vi "Helper Loop.vi"(8 "error in (no error)":errorcluster, 11 "Signal Analysis in":refnum<class "Signal Analysis.lvclass">) -> ()   [LabVIEW 2020, in "Signal Analysis.lvlib" / "Signal Analysis.lvclass"]
uses:
  Signal Analysis.lvclass
  C:/Program Files/National Instruments/LabVIEW 2025/vi.lib/ActorFramework/Actor/Actor.lvclass
  UI/UI Root/UI Root/Frequency Metadata.ctl
  Helper Loop State.ctl
  <vilib>/Natan Biesmans/G2CPU GPU and CPU HPC Toolkit/G2CPU Libraries/Arrays/1DArray/u32/1D Array u32.lvclass
  C:/Program Files/National Instruments/LabVIEW 2025/vi.lib/Natan Biesmans/G2CPU GPU and CPU HPC Toolkit/G2CPU Libraries/Arrays/Array/Array Prototype.lvclass
  <vilib>/Natan Biesmans/G2CPU GPU and CPU HPC Toolkit/G2CPU Libraries/Arrays/2DArray/s16/2D Array s16.lvclass
  <vilib>/Utility/miscctls.llb/LVOffsetAndMultiplierTypeDef.ctl
  Program Files/National Instruments/LabVIEW 2025/examples/Natan Biesmans/G2CPU GPU and CPU HPC Toolkit/_Examples/UI Acceleration/Signal Density Plot Config.ctl
  Signal Analysis.lvclass/Signal Analysis.ctl
  Helper Loop Message.ctl
  Helper Loop Type.ctl
  Process Data.ctl
  <vilib>/Natan Biesmans/G2CPU GPU and CPU HPC Toolkit/G2CPU Libraries/Arrays/1DArray/s16/1D Array s16.lvclass
  UI/UI Root/UI Root/Signal Density Plot Data.ctl
  UI/UI Root/UI Root/FFT Plot Data.ctl
  <vilib>/ActorFramework/Actor/Actor.lvclass/Actor.ctl
  Application Manager/Application Manager Messages/Visualize FFT Msg/Visualize FFT Msg.lvclass/Visualize FFT Msg.ctl
  <vilib>/ActorFramework/Message Enqueuer/Message Enqueuer.lvclass/Message Enqueuer.ctl
  Application Manager/Application Manager Messages/Update Processing Metrics Msg/Update Processing Metrics Msg.lvclass/Update Processing Metrics Msg.ctl
  FFT Size.ctl
  Low Prio Rendering.ctl
  3b7c5731-3288-422e-9579-54a588a7c3cc.vi
  5c8155d3-63a1-46d8-b807-fae1af1e600c.vi
  05f40b7a-0676-44ad-acd9-391c165d43ca.vi
  60a2c10f-7ea4-4c19-9847-04cfdb7c7b1d.vi
  b3cef79f-9c71-4781-96f4-977c5153f233.vi
  4c400397-ccdf-494a-85b7-b802f87979ea.vi
  e15d3b19-6d2e-4512-b034-1ccceea2a302.vi
  0b159706-0337-4146-9fcf-a9429f3d28bc.vi
  d3b2aca6-c04a-43a5-ac15-5dcc80cfe7fb.vi
  3b7c5731-3288-422e-9579-54a588a7c3cc.vi/6197f869-f6d4-49b3-9b2c-cc979b422c2e.vi
  3b7c5731-3288-422e-9579-54a588a7c3cc.vi/a7e86dbb-b4c0-485c-89c5-522e60ee265c.vi
  5c8155d3-63a1-46d8-b807-fae1af1e600c.vi/ff52a514-0e94-4685-9782-cee11f20a7e4.vi
  5c8155d3-63a1-46d8-b807-fae1af1e600c.vi/09f95493-deb6-40ba-ba08-e63bad1f3c71.vi
  05f40b7a-0676-44ad-acd9-391c165d43ca.vi/b1821858-f795-4172-8d77-0d2b0bdabb59.vi
  05f40b7a-0676-44ad-acd9-391c165d43ca.vi/d461e1dd-3ff8-4523-95b7-3ce56130f115.vi
  60a2c10f-7ea4-4c19-9847-04cfdb7c7b1d.vi/ef94ed2d-c4e6-48dc-8bdb-249d71a97973.vi
  b3cef79f-9c71-4781-96f4-977c5153f233.vi/ef94ed2d-c4e6-48dc-8bdb-249d71a97973.vi
  <vilib>/ActorFramework/Message Enqueuer/Enqueue.vi
  e15d3b19-6d2e-4512-b034-1ccceea2a302.vi/ab6cfe59-c8ad-4da3-839b-8d02ec9e015f.vi
  0b159706-0337-4146-9fcf-a9429f3d28bc.vi/46771f49-eb1d-473b-8e81-f516cef50a4e.vi
  0b159706-0337-4146-9fcf-a9429f3d28bc.vi/dc76f8e4-64fa-456a-8549-7a4b6936c4c9.vi
  0b159706-0337-4146-9fcf-a9429f3d28bc.vi/7e60ddfb-e748-4c0c-85da-e395a1b7978d.vi
  0b159706-0337-4146-9fcf-a9429f3d28bc.vi/d2eceff7-f641-4ce4-acfa-e9e293a3c877.vi
  0b159706-0337-4146-9fcf-a9429f3d28bc.vi/b737122b-4036-448b-abd3-e2701355e828.vi
  d3b2aca6-c04a-43a5-ac15-5dcc80cfe7fb.vi/e7247370-a01f-465a-ac0e-4dfefcb1bb87.vi
  d3b2aca6-c04a-43a5-ac15-5dcc80cfe7fb.vi/345e91f0-9a5e-4de4-af9c-133346717e4a.vi
  3b7c5731-3288-422e-9579-54a588a7c3cc.vi/6197f869-f6d4-49b3-9b2c-cc979b422c2e.vi/87b81512-7a6a-4bb0-93b2-4564eba18751.vi
  3b7c5731-3288-422e-9579-54a588a7c3cc.vi/6197f869-f6d4-49b3-9b2c-cc979b422c2e.vi/3b85cfcd-f2e7-425d-bf63-d84251333cff.vi
  3b7c5731-3288-422e-9579-54a588a7c3cc.vi/6197f869-f6d4-49b3-9b2c-cc979b422c2e.vi/bdde7ba0-fc5a-4512-a8ec-1695e5fcee25.vi
  3b7c5731-3288-422e-9579-54a588a7c3cc.vi/6197f869-f6d4-49b3-9b2c-cc979b422c2e.vi/3e802c67-fb96-46a3-ae13-4994a8508b4f.vi
  3b7c5731-3288-422e-9579-54a588a7c3cc.vi/6197f869-f6d4-49b3-9b2c-cc979b422c2e.vi/5a50fc67-79e7-4972-80c2-92243cd53dd4.vi
  3b7c5731-3288-422e-9579-54a588a7c3cc.vi/a7e86dbb-b4c0-485c-89c5-522e60ee265c.vi/730f6c57-5c0b-4ee9-b61e-75067b25222b.vi
  3b7c5731-3288-422e-9579-54a588a7c3cc.vi/a7e86dbb-b4c0-485c-89c5-522e60ee265c.vi/096b8799-7810-404e-baca-ba9279cec4bd.vi
  3b7c5731-3288-422e-9579-54a588a7c3cc.vi/a7e86dbb-b4c0-485c-89c5-522e60ee265c.vi/0f1a5a47-bcc5-4796-ac31-8dfcfbc0d7d1.vi
  3b7c5731-3288-422e-9579-54a588a7c3cc.vi/a7e86dbb-b4c0-485c-89c5-522e60ee265c.vi/89f12e17-3330-4b72-ad8f-8dd636660732.vi
  e15d3b19-6d2e-4512-b034-1ccceea2a302.vi/ab6cfe59-c8ad-4da3-839b-8d02ec9e015f.vi/313ec8c5-c203-475c-9de0-0583f6fb8b4d.vi
  0b159706-0337-4146-9fcf-a9429f3d28bc.vi/dc76f8e4-64fa-456a-8549-7a4b6936c4c9.vi/2c12aba4-aacf-4d7a-adbe-039f6155a93e.vi
  0b159706-0337-4146-9fcf-a9429f3d28bc.vi/dc76f8e4-64fa-456a-8549-7a4b6936c4c9.vi/f38cccb2-46f6-49f0-a8d6-9da0c88ff6f3.vi
  0b159706-0337-4146-9fcf-a9429f3d28bc.vi/dc76f8e4-64fa-456a-8549-7a4b6936c4c9.vi/bdde7ba0-fc5a-4512-a8ec-1695e5fcee25.vi
  0b159706-0337-4146-9fcf-a9429f3d28bc.vi/dc76f8e4-64fa-456a-8549-7a4b6936c4c9.vi/3e802c67-fb96-46a3-ae13-4994a8508b4f.vi
  0b159706-0337-4146-9fcf-a9429f3d28bc.vi/dc76f8e4-64fa-456a-8549-7a4b6936c4c9.vi/5a50fc67-79e7-4972-80c2-92243cd53dd4.vi
  3b7c5731-3288-422e-9579-54a588a7c3cc.vi/6197f869-f6d4-49b3-9b2c-cc979b422c2e.vi/3e802c67-fb96-46a3-ae13-4994a8508b4f.vi/1b7cf390-2ae0-48f3-9bce-03c57eed6ee8.vi
  0b159706-0337-4146-9fcf-a9429f3d28bc.vi/dc76f8e4-64fa-456a-8549-7a4b6936c4c9.vi/5a50fc67-79e7-4972-80c2-92243cd53dd4.vi/1b7cf390-2ae0-48f3-9bce-03c57eed6ee8.vi
  <vilib>/Natan Biesmans/G2CPU GPU and CPU HPC Toolkit/G2CPU Libraries/Arrays/1DArray/f32/1D Array f32.lvclass
  <vilib>/Natan Biesmans/G2CPU GPU and CPU HPC Toolkit/G2CPU Libraries/Arrays/2DArray/c32/2D Array c32.lvclass
  <vilib>/Natan Biesmans/G2CPU GPU and CPU HPC Toolkit/G2CPU Libraries/Arrays/2DArray/f32/2D Array f32.lvclass
  Application Manager/Application Manager Messages/Visualize FFT Msg/Visualize FFT Msg.lvclass
  C:/Program Files/National Instruments/LabVIEW 2025/vi.lib/ActorFramework/Message/Message.lvclass
  Application Manager/Application Manager Messages/Update Processing Metrics Msg/Update Processing Metrics Msg.lvclass
  <vilib>/Natan Biesmans/G2CPU GPU and CPU HPC Toolkit/G2CPU Libraries/Arrays/1DArray/u64/1D Array u64.lvclass
  <vilib>/Natan Biesmans/G2CPU GPU and CPU HPC Toolkit/ArrayFire Driver/VIs/Run as Multi Device.vi
  <vilib>/Natan Biesmans/G2CPU GPU and CPU HPC Toolkit/G2CPU Libraries/Manage Environment/Find AF DLL.vi
  <vilib>/Natan Biesmans/G2CPU GPU and CPU HPC Toolkit/ArrayFire Driver/subvi/Error Converter (ErrCode or Status).vi
  <vilib>/Natan Biesmans/G2CPU GPU and CPU HPC Toolkit/G2CPU Libraries/Arrays/Array/G2CPU Set Array Pointer.vi
  <vilib>/Natan Biesmans/G2CPU GPU and CPU HPC Toolkit/G2CPU Libraries/Arrays/Array/G2CPU Get Array Pointer.vi
  <vilib>/Natan Biesmans/G2CPU GPU and CPU HPC Toolkit/ArrayFire Driver/VIs/cast.vi
  <vilib>/Natan Biesmans/G2CPU GPU and CPU HPC Toolkit/G2CPU Libraries/Arrays/SubVI/Lock Arrays.vi
  <vilib>/Natan Biesmans/G2CPU GPU and CPU HPC Toolkit/G2CPU Libraries/Arrays/SubVI/is 2D.vi
  <vilib>/Natan Biesmans/G2CPU GPU and CPU HPC Toolkit/ArrayFire Driver/VIs/mul.vi
  <vilib>/Natan Biesmans/G2CPU GPU and CPU HPC Toolkit/G2CPU Libraries/Arrays/Array/G2CPU Unlock Array.vi
  <vilib>/Natan Biesmans/G2CPU GPU and CPU HPC Toolkit/ArrayFire Driver/VIs/fft inplace.vi
  <vilib>/Natan Biesmans/G2CPU GPU and CPU HPC Toolkit/ArrayFire Driver/VIs/max by key.vi
  <vilib>/Natan Biesmans/G2CPU GPU and CPU HPC Toolkit/G2CPU Libraries/Arrays/Array/G2CPU Get Array Size.vi
  <vilib>/Natan Biesmans/G2CPU GPU and CPU HPC Toolkit/G2CPU Libraries/Arrays/Array/G2CPU Get Data Type.vi
  <vilib>/Natan Biesmans/G2CPU GPU and CPU HPC Toolkit/ArrayFire Driver/VIs/is scalar.vi
  <vilib>/Natan Biesmans/G2CPU GPU and CPU HPC Toolkit/ArrayFire Driver/VIs/is empty.vi
  <vilib>/ActorFramework/Message Priority Queue/Priority Enqueue.vi
  <vilib>/Natan Biesmans/G2CPU GPU and CPU HPC Toolkit/ArrayFire Driver/VIs/range.vi
  <vilib>/Natan Biesmans/G2CPU GPU and CPU HPC Toolkit/G2CPU Libraries/Arrays/SubVI/is 1D.vi
  <vilib>/Natan Biesmans/G2CPU GPU and CPU HPC Toolkit/ArrayFire Driver/VIs/div.vi
  <vilib>/Natan Biesmans/G2CPU GPU and CPU HPC Toolkit/G2CPU Libraries/Arrays/Array/Array Prototype.lvclass
  <vilib>/Natan Biesmans/G2CPU GPU and CPU HPC Toolkit/G2CPU Libraries/Arrays/DataTypes/c32/c32.lvclass
  <vilib>/Natan Biesmans/G2CPU GPU and CPU HPC Toolkit/G2CPU Libraries/Arrays/2DArray/2D Array Prototype.lvclass
  <vilib>/Natan Biesmans/G2CPU GPU and CPU HPC Toolkit/G2CPU Libraries/Arrays/DataTypes/f32/f32.lvclass
  <vilib>/Natan Biesmans/G2CPU GPU and CPU HPC Toolkit/G2CPU Libraries/Arrays/1DArray/1D Array Prototype.lvclass
  <vilib>/ptbypt/NI_PtbyPt.lvlib
  <vilib>/Natan Biesmans/G2CPU GPU and CPU HPC Toolkit/G2CPU Libraries/UI Acceleration/G2CPU Signal Density Plots.lvlib
  UI/UI Root/UI Root/UI Root.lvclass
  <vilib>/ActorFramework/Actor/Actor.lvclass
panel:
  in  "Frequency Metedata":T1
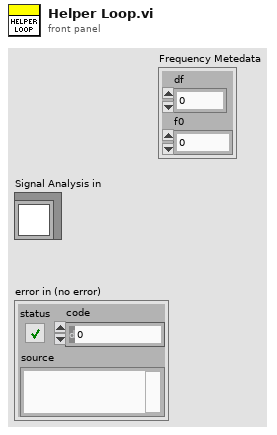
[diagram p1: front panel]
types:
  T1 = typedef "UI Root.lvlib/UI Root.lvclass/Frequency Metadata.ctl" = cluster{"df":dbl, "f0":dbl}
  T2 = typedef "Signal Analysis.lvlib/Signal Analysis.lvclass/Helper Loop State.ctl" = cluster{"First Run":bool, "Plot Scale":cluster{"X Scale":T3, "Y Scale":T3}, "Predefined Configuration Parameters":cluster{"Column Counter":refnum<class "1D Array u32.lvclass">, "Full Bin Range":refnum<class "2D Array s16.lvclass">}, "FFT Size":i32, "Low Prio Rendering":bool, "FFT Scaling Map":refnum<class "1D Array u32.lvclass">, "FFT Scaling":dbl, "Graph Config":T4}
  T3 = typedef "LVOffsetAndMultiplierTypeDef.ctl" = cluster{"Offset":dbl, "Multiplier":dbl}
  T4 = typedef "G2CPU Signal Density Plots.lvlib/Signal Density Plot Config.ctl" = cluster{"X resolution":u64, "Y resolution":u64, "Min":sgl, "Max":sgl}
  T5 = typedef "UI Root.lvlib/UI Root.lvclass/FFT Plot Data.ctl" = cluster{"FFT":refnum<data-value>, "Scaling":dbl, "Raw FFT Size":i32}
  T6 = typedef "UI Root.lvlib/UI Root.lvclass/Signal Density Plot Data.ctl" = cluster{"Plot":refnum<data-value>, "Plot Scale":cluster{"X Scale":T3, "Y Scale":T3}}
  T7 = typedef "Signal Analysis.lvlib/Signal Analysis.lvclass/Process Data.ctl" = cluster{"Gain":dbl, "dt":dbl, "Serial IQ Data":refnum<class "1D Array s16.lvclass">, "f0":dbl}
  T8 = typedef "Signal Analysis.lvlib/Signal Analysis.lvclass/FFT Size.ctl" = cluster{"FFT Size":i32}
  T9 = typedef "Signal Analysis.lvlib/Signal Analysis.lvclass/Low Prio Rendering.ctl" = cluster{"Low Prio Rendering":bool}
  T10 = typedef "Signal Analysis.lvlib/Signal Analysis.lvclass/Helper Loop Message.ctl" = cluster{"Type":T11, "Payload":variant}
  T11 = typedef "Signal Analysis.lvlib/Signal Analysis.lvclass/Helper Loop Type.ctl" = enum16{"Process Data", "Set Batch Size", "Set Render Prio", "Close", "Set FFT Size"}
  T12 = cluster{"Column Counter":refnum<class "1D Array u32.lvclass">, "Full Bin Range":refnum<class "2D Array s16.lvclass">}
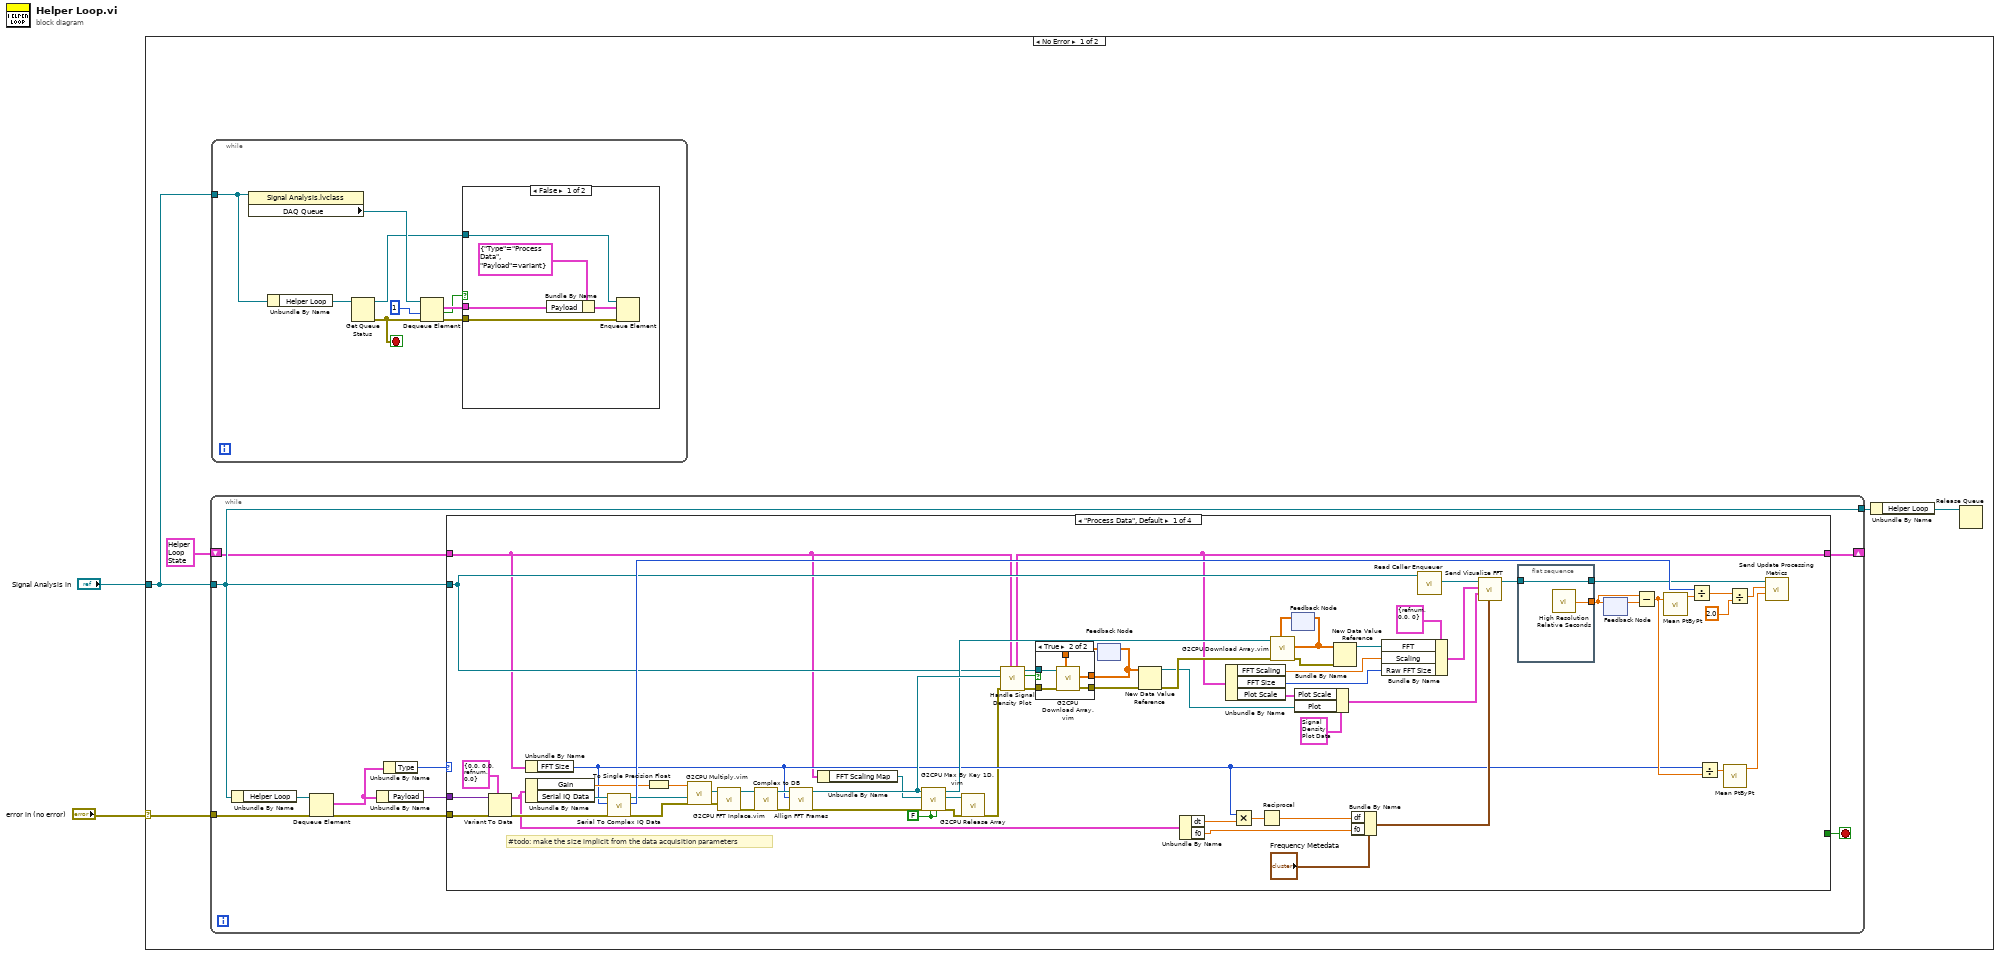
[diagram p0: block diagram]
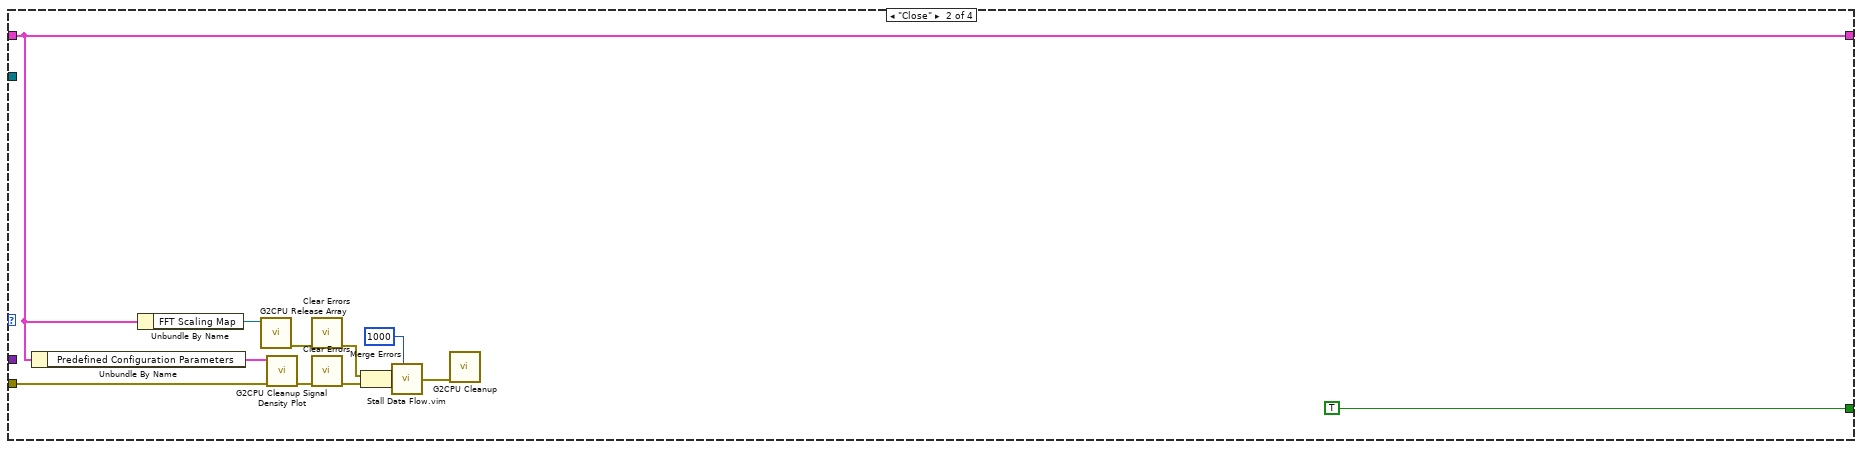
[diagram p3: hidden frame]
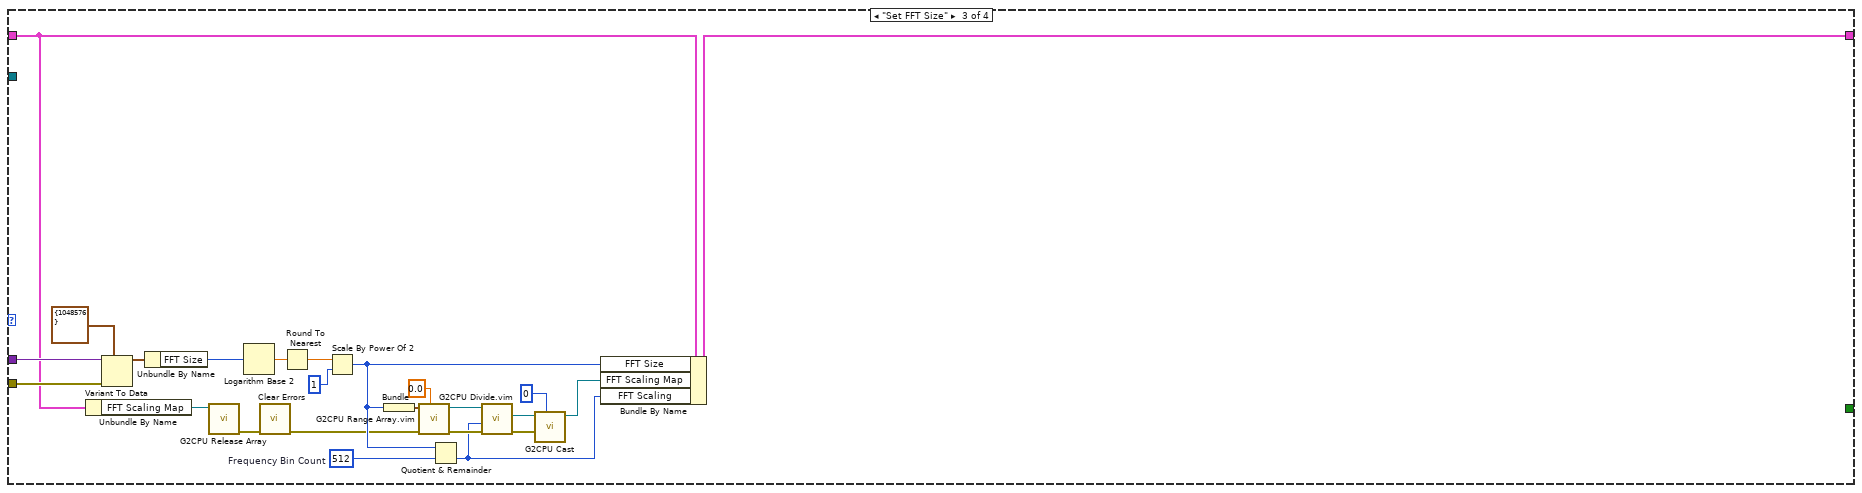
[diagram p4: hidden frame]
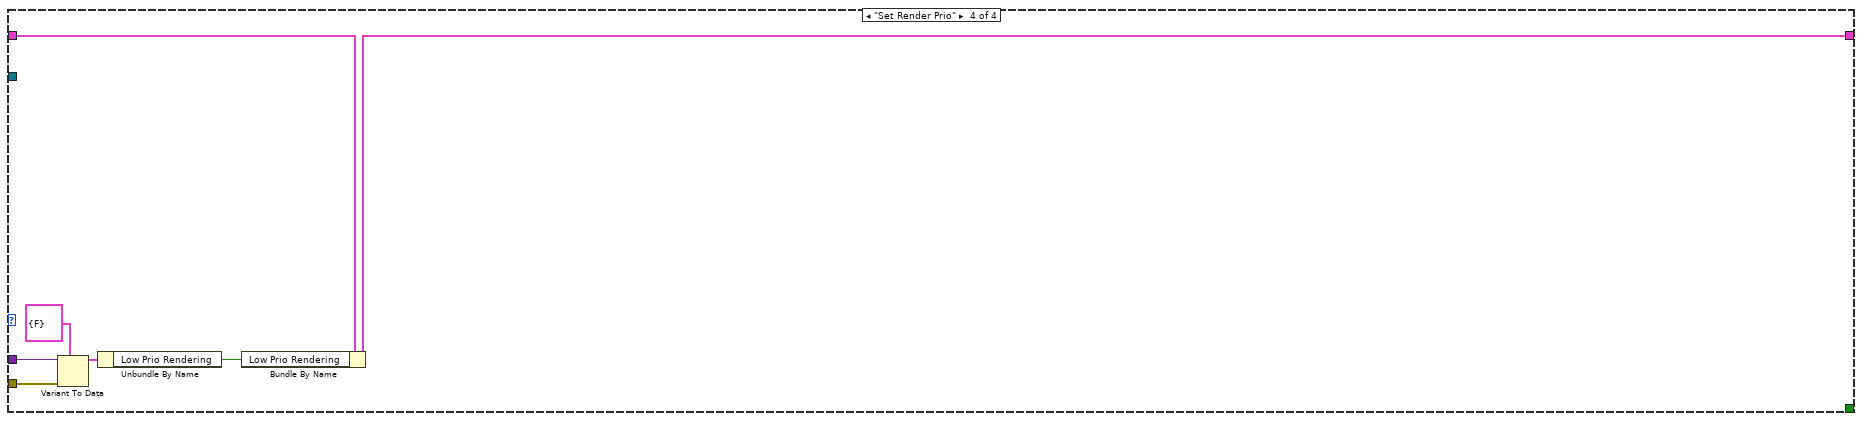
[diagram p5: hidden frame]
diagram:
  n1 = case shown="No Error" "error in (no error)" {
    selector: "error in (no error)" -> [w7 _]
    tunnel: "Signal Analysis in" -> [w6 _]
    frame No Error {
      n2 = while {
        tunnel: w6 -> [w12]
        tunnel: w7 -> [w17]
        tunnel: [w12] -> w5
        shift-right: [w9] -> _
        shift-left: T2 {"First Run"=TRUE, "Plot Scale"={"X Scale"={"Offset"=0.0, "Multiplier"=0.0}, "Y Scale"={"Offset"=0.0, "Multiplier"=0.0}}, "Predefined Configuration Parameters"={"Column Counter"=refnum, "Full Bin Range"=refnum}, "FFT Size"=1048576, "Low Prio Rendering"=FALSE, "FFT Scaling Map"=refnum, "FFT Scaling"=0.0, "Graph Config"={"X resolution"=0, "Y resolution"=0, "Min"=0.0, "Max"=0.0}} ("State") -> [w8]
        stop <- w14 stop-if-true
        n3 = Unbundle By Name(w12) -> ("Helper Loop"=w16:refnum<queue>)
        n4 = Dequeue Element(queue=w16, error in (no error)=w17) -> (element=w13:T10, error out=w15:errorcluster)  [unwired: 1 in, 2 out]
        n5 = Unbundle By Name(w13) -> ("Payload"=w10:variant)
        n6 = Unbundle By Name(w13) -> ("Type"=w11:T11)
        n7 = case shown="\"Process Data\", Default" w11 {
          tunnel: w12 -> [w40 _ _ _]
          tunnel: w15 -> [w83 w103 w126 w134]
          tunnel: [_ TRUE _ _] -> w14
          tunnel: w10 -> [w82 _ w127 w133]
          tunnel: [w30 w95 w128 w131] -> w9
          tunnel: w8 -> [w31 w95 w110 w135]
          frame "Process Data", Default {
            w36 = FALSE ("Auto Release Keys (Enabled)")
            # "#todo: make the size implicit from the data acquisition parameters"
            n8 = Variant To Data(error in=w83, type=T7 {"Gain"=0.0, "dt"=0.0, "Serial IQ Data"=refnum, "f0"=0.0} ("Filled Buffers"), Variant=w82) -> (data=w50:T7, error out=w81:errorcluster)
            n9 = Unbundle By Name(w50) -> ("Gain"=w56:dbl, "Serial IQ Data"=w61:refnum<class "1D Array s16.lvclass">)
            n10 = Unbundle By Name(w31) -> ("FFT Size"=w39:i32)
            n11 = call "Serial To Complex IQ Data.vi"("error in (no error)"=w81, "FFT Size"=w39, "Serial Data In"=w61) -> ("error out"=w53:errorcluster, "Amount Of Samples"=w74:u64, "Batched Complex Data Out"=w55:refnum<class "2D Array c32.lvclass">)  [unwired: 5 in, 1 out]
            n12 = To Single Precision Float(number=w56) -> (single precision float=w54:sgl)
            n13 = call "G2CPU Multiply.vim"("error in (no error)"=w53, "Array rhs"=w55, "Array lhs"=w54) -> ("error out"=w52:errorcluster, "Array Result"=w51:refnum<class "2D Array c32.lvclass">)  [unwired: 7 in]
            n14 = call "G2CPU FFT Inplace.vim"("error in (no error)"=w52, "Array Signal"=w51) -> ("error out"=w57:errorcluster, "Array out"=w58:refnum<class "2D Array c32.lvclass">)  [unwired: 8 in]
            n15 = call "Complex to DB.vi"("error in (no error)"=w57, "Complix FFT In"=w58) -> ("error out"=w59:errorcluster, "Db Amplitude Out"=w60:refnum<class "2D Array f32.lvclass">)  [unwired: 8 in]
            n16 = call "Allign FFT Frames.vi"("error in (no error)"=w59, "FFT Size"=w39, "FFT Frame in"=w60) -> ("error out"=w38:errorcluster, "Alligned FFT Frame Out"=w65:refnum<class "2D Array f32.lvclass">)  [unwired: 6 in, 1 out]
            n17 = Unbundle By Name(w31) -> ("FFT Scaling Map"=w37:refnum<class "1D Array u32.lvclass">)
            n18 = call "G2CPU Max By Key 1D.vim"("Auto Release Keys (Enabled)"=w36, "Auto Release Array In (Enabled)"=w36, "error in (no error)"=w38, "Array Keys 1D U32"=w37, "Array"=w65) -> ("error out"=w79:errorcluster, "Array Keys"=w80:refnum<class "1D Array u32.lvclass">, "Array out"=w41:refnum<class "2D Array f32.lvclass">)  [unwired: 4 in]
            n19 = call <vilib>:"G2CPU Release Array.vi"("error in (no error)"=w79, "Array in"=w80) -> ("error out"=w32:errorcluster)  [unwired: 9 in]
            n20 = call "Handle Signal Density Plot.vi"("State in"=w31, "error in (no error)"=w32, "Alligned FFT Frame Out"=w65, "Signal Analysis in"=w40) -> ("error out"=w70:errorcluster, "Signal Density Plot Available"=w29:bool, "Signal Density Plot"=w69:refnum<class "2D Array f32.lvclass">, "State out"=w30:T2)  [unwired: 4 in]
            n21 = feedback #1() -> (w68:sgl[][])  [unwired: 1 in]
            n22 = case shown="True" w29 {
              tunnel: w70 -> [w86 w92]
              tunnel: w69 -> [_ w91]
              tunnel: w68 -> [w87 w90]
              tunnel: [w86 w89] -> w67
              tunnel: [w87 w88] -> w66
              frame False {
              }
              frame True {
                n23 = call "G2CPU Download Array.vim"("Pre Allocated Buffer"=w90, "error in (no error)"=w92, "Array in"=w91) -> ("error out"=w89:errorcluster, "Array Data"=w88:sgl[][])  [unwired: 6 in, 1 out]
              }
            }
            n24 = feedback-in #1(w66) -> ()
            n25 = New Data Value Reference(data value=w66, error in=w67) -> (data value reference=w28:refnum<data-value>, error out=w42:errorcluster)
            n26 = Unbundle By Name(w50) -> ("dt"=w49:dbl, "f0"=w33:dbl)
            n27 = Unbundle By Name(w30) -> ("FFT Scaling"=w35:dbl, "FFT Size"=w34:i32, "Plot Scale"=w27:cluster{"X Scale":T3, "Y Scale":T3})
            n28 = Multiply(x=w39, y=w49) -> (x*y=w44:dbl)
            n29 = Reciprocal(x=w44) -> (1/x=w43:dbl)
            n30 = feedback #2() -> (w26:sgl[][])  [unwired: 1 in]
            n31 = call "G2CPU Download Array.vim"("Pre Allocated Buffer"=w26, "error in (no error)"=w42, "Array in"=w41) -> ("error out"=w21:errorcluster, "Array Data"=w25:sgl[][])  [unwired: 6 in, 1 out]
            n32 = feedback-in #2(w25) -> ()
            n33 = Bundle By Name(cluster=T6 {"Plot"=refnum, "Plot Scale"={"X Scale"={"Offset"=0.0, "Multiplier"=0.0}, "Y Scale"={"Offset"=0.0, "Multiplier"=0.0}}} ("output cluster 2"), "Plot Scale"=w27, "Plot"=w28) -> (w47:T6)
            n34 = New Data Value Reference(data value=w25, error in=w21) -> (data value reference=w22:refnum<data-value>)  [unwired: 1 out]
            n35 = Bundle By Name(cluster="Frequency Metedata", "df"=w43, "f0"=w33) -> (w45:T1)
            n36 = Bundle By Name(cluster=T5 {"FFT"=refnum, "Scaling"=0.0, "Raw FFT Size"=0} ("FFT Data"), "FFT"=w22, "Scaling"=w35, "Raw FFT Size"=w34) -> (w23:T5)
            n37 = call <vilib>:"Read Caller Enqueuer.vi"("Actor"=w40) -> ("Caller Enqueuer"=w20:refnum<class "Message Enqueuer.lvclass">)  [unwired: 10 in]
            n38 = call "Send Visualize FFT.vi"("Frequency Metedata"=w45, "Signal Density Plot"=w47, "FFT Data"=w23, "Message Enqueuer"=w20) -> ("Message Enqueuer out"=w19:refnum<class "Message Enqueuer.lvclass">)  [unwired: 6 in, 1 out]
            n39 = flat-sequence {
              tunnel: [w85] -> w77
              tunnel: [w84] -> w18
              tunnel: w19 -> [w84]
              frame #0 {
                n40 = call <vilib>:"High Resolution Relative Seconds.vi"() -> ("relative seconds"=w85:dbl)
              }
            }
            n41 = feedback #3() -> (w78:dbl)  [unwired: 1 in]
            n42 = feedback-in #3(w77) -> ()
            n43 = Subtract(x=w77, y=w78) -> (x-y=w72:dbl)
            n44 = call <vilib>:"Mean PtByPt.vi"("x"=w72) -> ("mean"=w76:dbl)  [unwired: 3 in, 1 out]
            n45 = Divide(x=w74, y=w76) -> (x/y=w75:dbl)
            n46 = Divide(x=w39, y=w72) -> (x/y=w71:dbl)
            n47 = call <vilib>:"Mean PtByPt.vi"("x"=w71) -> ("mean"=w64:dbl)  [unwired: 3 in, 1 out]
            n48 = Divide(x=w75, y=2.0) -> (x/y=w63:dbl)
            n49 = call "Send Update Processing Metrics.vi"("Peak Output"=w64, "System Throughput"=w63, "Message Enqueuer"=w18) -> ()  [unwired: 7 in, 2 out]
          }
          frame "Close" {
            n50 = Unbundle By Name(w95) -> ("Predefined Configuration Parameters"=w98:T12)
            n51 = Unbundle By Name(w95) -> ("FFT Scaling Map"=w97:refnum<class "1D Array u32.lvclass">)
            n52 = call <vilib>:"G2CPU Release Array.vi"("Array in"=w97) -> ("error out"=w96:errorcluster)  [unwired: 10 in]
            n53 = call <vilib>:"G2CPU Cleanup Signal Density Plot.vi"("error in (no error)"=w103, "Predefined Configuration Parameters"=w98) -> ("error out"=w100:errorcluster)  [unwired: 9 in]
            n54 = call <vilib>:"Clear Errors.vi"("error in (no error)"=w96) -> ("error out"=w93:errorcluster)  [unwired: 5 in, 1 out]
            n55 = call <vilib>:"Clear Errors.vi"("error in (no error)"=w100) -> ("error out"=w99:errorcluster)  [unwired: 5 in, 1 out]
            n56 = Merge Errors(w93, w99) -> (w94:errorcluster)
            n57 = call "Stall Data Flow.vim"("value in"=w94, "milliseconds to wait"=u32 1000) -> ("value out"=w102:errorcluster)  [unwired: 1 out]
            n58 = call <vilib>:"G2CPU Cleanup.vi"("error in (no error)"=w102) -> ()  [unwired: 10 in, 1 out]
          }
          frame "Set FFT Size" {
            w106 = u64 512  # Frequency Bin Count
            n59 = Unbundle By Name(w110) -> ("FFT Scaling Map"=w109:refnum<class "1D Array u32.lvclass">)
            n60 = Variant To Data(error in=w126, type=T8 {"FFT Size"=1048576} ("FFT Size"), Variant=w127) -> (data=w124:T8)  [unwired: 1 out]
            n61 = Unbundle By Name(w124) -> ("FFT Size"=w120:i32)
            n62 = call <vilib>:"G2CPU Release Array.vi"("Array in"=w109) -> ("error out"=w108:errorcluster)  [unwired: 10 in]
            n63 = Logarithm Base 2(1:w120) -> (0:w123:dbl)
            n64 = call <vilib>:"Clear Errors.vi"("error in (no error)"=w108) -> ("error out"=w107:errorcluster)  [unwired: 5 in, 1 out]
            n65 = Round To Nearest(number=w123) -> (nearest integer value=w122:dbl)
            n66 = Scale By Power Of 2(n=w122, x=u64 1) -> (x*2^n=w112:u64)
            n67 = Bundle(w112) -> (w119:cluster{u64})  [unwired: 1 in]
            n68 = call "G2CPU Range Array.vim"("Datatype"=sgl 0.0, "Error in"=w107, "Size"=w119) -> ("error out"=w116:errorcluster, "Array out"=w115:refnum<class "1D Array f32.lvclass">)  [unwired: 7 in]
            n69 = Quotient & Remainder(x=w112, y=w106) -> (floor(x/y)=w105:u64)  [unwired: 1 out]
            n70 = call "G2CPU Divide.vim"("error in (no error)"=w116, "Array rhs"=w105, "Array lhs"=w115) -> ("error out"=w118:errorcluster, "Array Result"=w117:refnum<class "1D Array f32.lvclass">)  [unwired: 7 in]
            n71 = call "G2CPU Cast"("Datatype Prototype"=u32 0, "error in (no error)"=w118, "Array In"=w117) -> ("Array Out"=w111:refnum<class "1D Array u32.lvclass">)  [unwired: 7 in, 1 out]
            n72 = Bundle By Name(cluster=w110, "FFT Size"=w112, "FFT Scaling Map"=w111, "FFT Scaling"=w105) -> (w128:T2)
          }
          frame "Set Render Prio" {
            n73 = Variant To Data(error in=w134, type=T9 {"Low Prio Rendering"=FALSE} ("Low Prio Rendering"), Variant=w133) -> (data=w130:T9)  [unwired: 1 out]
            n74 = Unbundle By Name(w130) -> ("Low Prio Rendering"=w129:bool)
            n75 = Bundle By Name(cluster=w135, "Low Prio Rendering"=w129) -> (w131:T2)
          }
        }
      }
      n76 = while {
        tunnel: w6 -> [w139]
        stop <- w138 stop-if-true
        n77 = property class="Signal Analysis.lvclass"(reference=w139) -> ("DAQ Queue"=w140:refnum<queue>)  [unwired: 1 in, 2 out]
        n78 = Unbundle By Name(w139) -> ("Helper Loop"=w137:refnum<queue>)
        n79 = Get Queue Status(queue=w137) -> (queue out=w136:refnum<queue>, error out=w138:errorcluster)  [unwired: 2 in, 6 out]
        n80 = Dequeue Element(queue=w140, timeout in ms (-1)=1, error in (no error)=w138) -> (element=w144:T7, timed out?=w143:bool, error out=w142:errorcluster)  [unwired: 1 out]
        n81 = case shown="False" w143 {
          tunnel: w142 -> [w148 _]
          tunnel: w144 -> [w145 _]
          tunnel: w136 -> [w149 _]
          frame False {
            n82 = Bundle By Name(cluster=T10 {"Type"=enum."Process Data", "Payload"=variant} ("element"), "Payload"=w145) -> (w146:T10)
            n83 = Enqueue Element(queue=w149, element=w146, error in (no error)=w148) -> ()  [unwired: 1 in, 3 out]
          }
          frame True {
          }
        }
      }
      n84 = Unbundle By Name(w5) -> ("Helper Loop"=w4:refnum<queue>)
      n85 = Release Queue(queue=w4) -> ()  [unwired: 2 in, 3 out]
    }
    frame Error {
    }
  }
